vi "Error Invalid ASE Handle.vi"() -> (0 "Invalid ASE Handle":errorcluster)   [LabVIEW 2020, in "ase.lvlib" / "ase.lvclass"]
doc: "Error constant"
uses:
  ase.lvclass
  ase.lvclass/ase.ctl
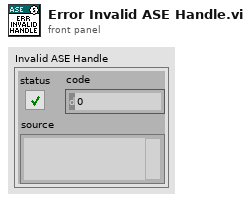
[diagram p1: front panel]
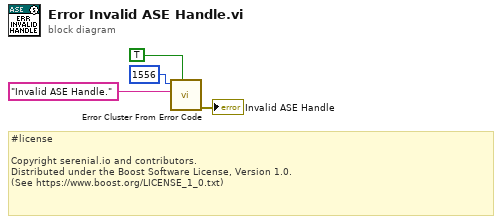
[diagram p0: block diagram]
diagram:
  # "#license\n\nCopyright serenial.io and contributors.\nDistributed under the Boost Software License, Version 1.0.\n(See https://www.boost.org/LICENSE_1_0.txt)"
  n1 = call <vilib>:"Error Cluster From Error Code.vi"("show call chain? (False)"=TRUE, "error message (\"\")"="Invalid ASE Handle." ("error message (\"\")"), "error code (0)"=1556) -> ("error out"=→"Invalid ASE Handle":errorcluster)  [unwired: 6 in]
